vi "Info.vi"(9 "deutsch?":bool, 10 "virsualisierung?":bool, 11 "Version":string) -> ()   [LabVIEW 2012]
panel:
  in  "ende?":bool
  out "Numerisch":i32
  out "2D-Bild":picture
  out "Fehler (Ausgang)":errorcluster
  out "OK-Schaltfläche":bool
  # "2009 - 2011"
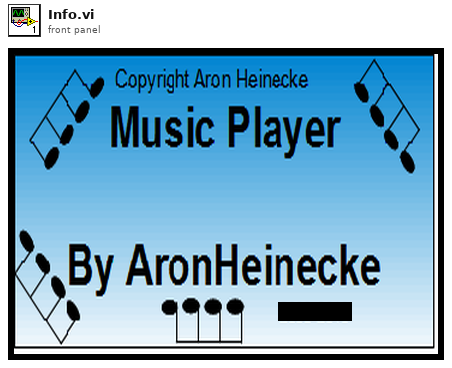
[diagram p1: front panel]
types:
  T1 = enum16{"None", "Stacked", "Clockwise", "Counterclockwise"}
  T2 = cluster{"Font Name:":string, "Size":i16, "Strikeout?":bool, "Italic?":bool, "Underline?":bool, "Outline?":bool, "Shadow?":bool, "Bold?":bool}
  T3 = cluster{"horizontal":enum16{"left", "center", "right"}, "vertical":enum16{"top", "center", "bottom"}}
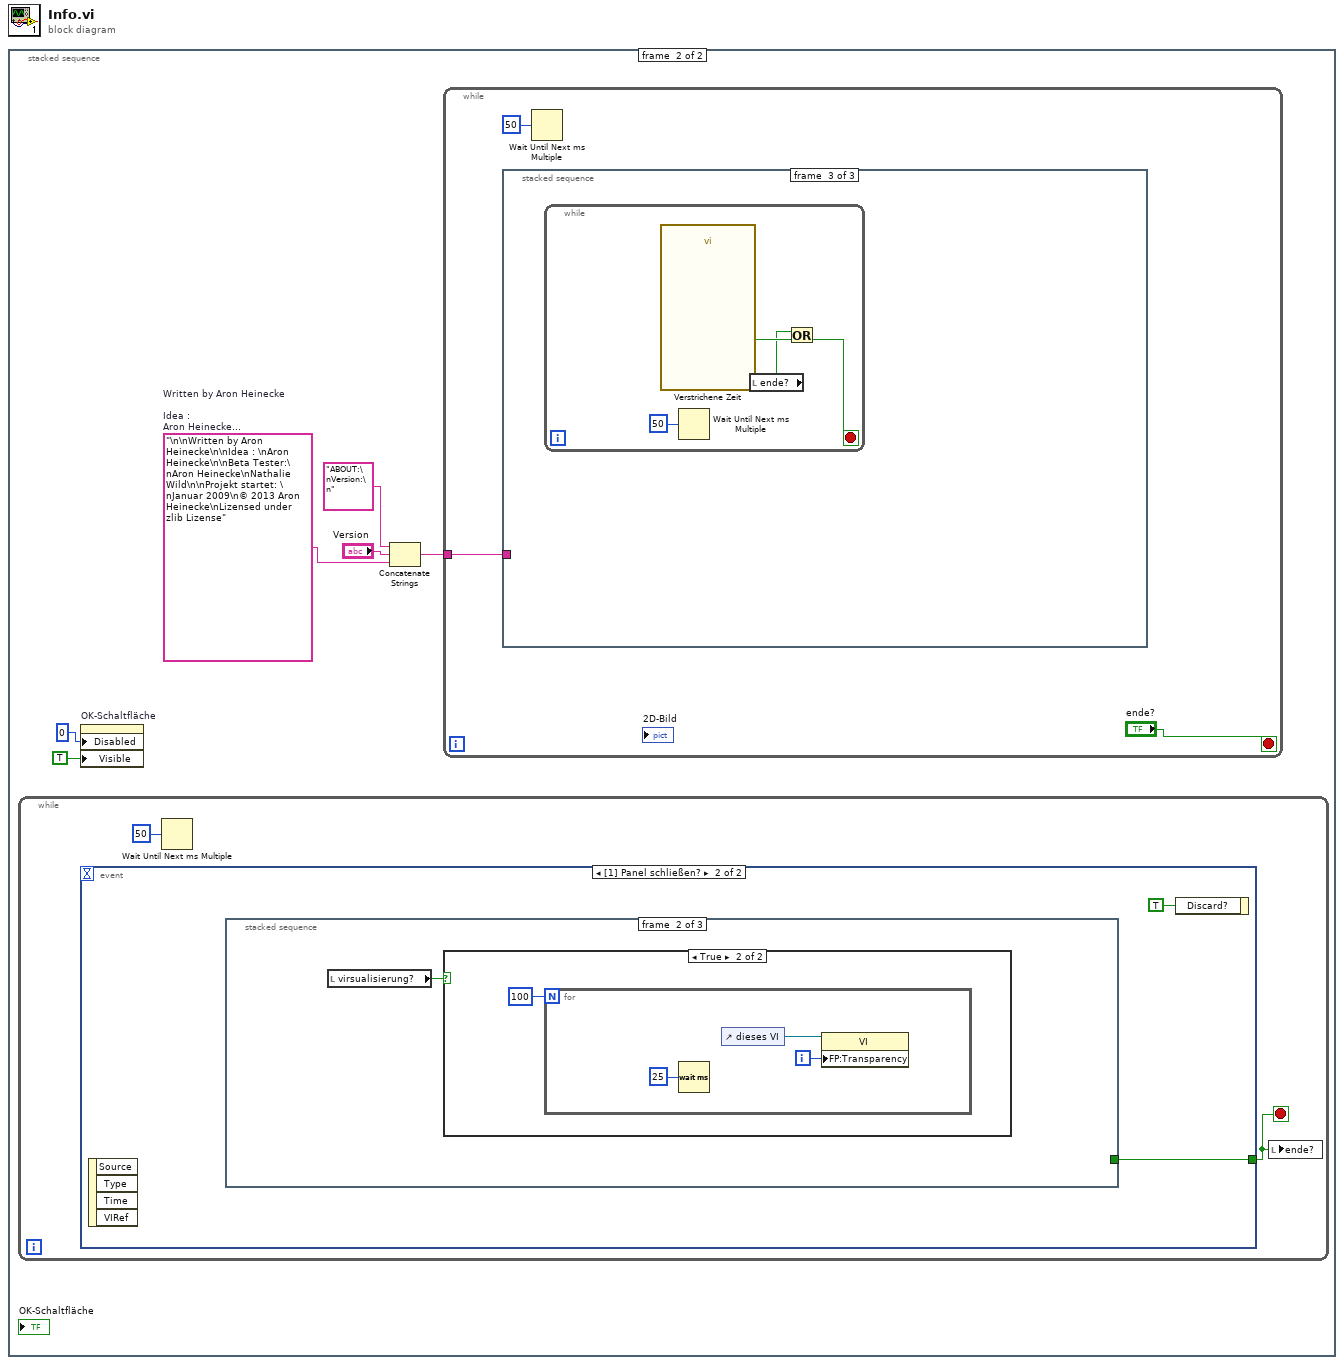
[diagram p0: block diagram]
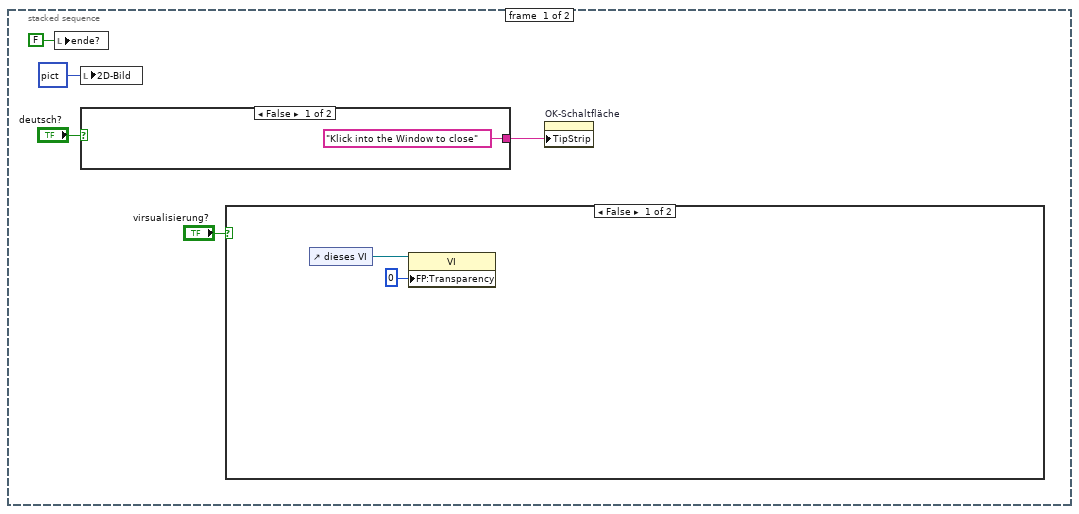
[diagram p2: hidden frame]
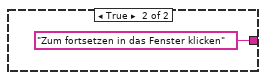
[diagram p3: hidden frame]
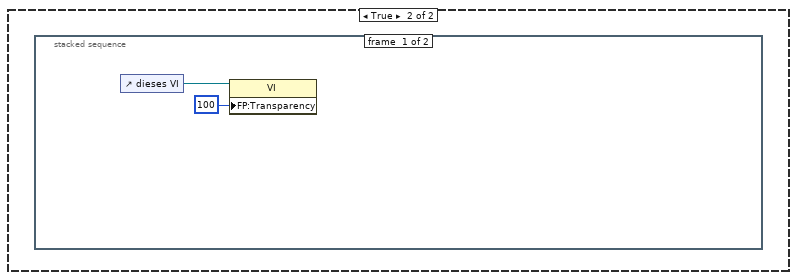
[diagram p4: hidden frame]
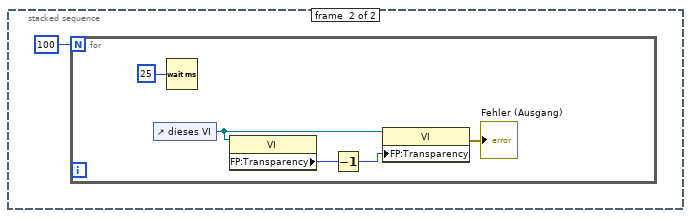
[diagram p5: hidden frame]
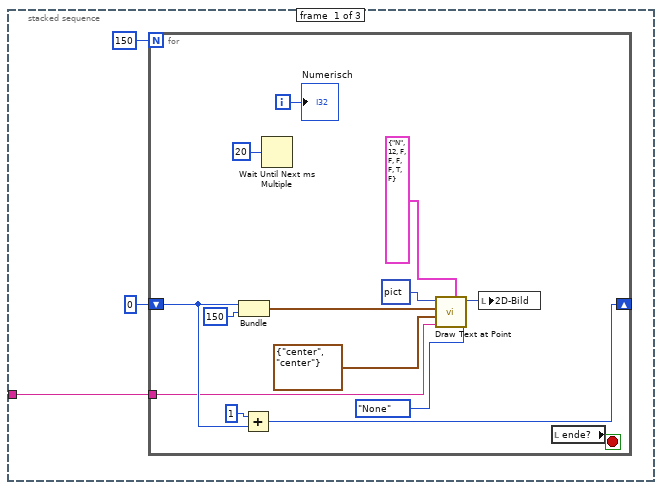
[diagram p6: hidden frame]
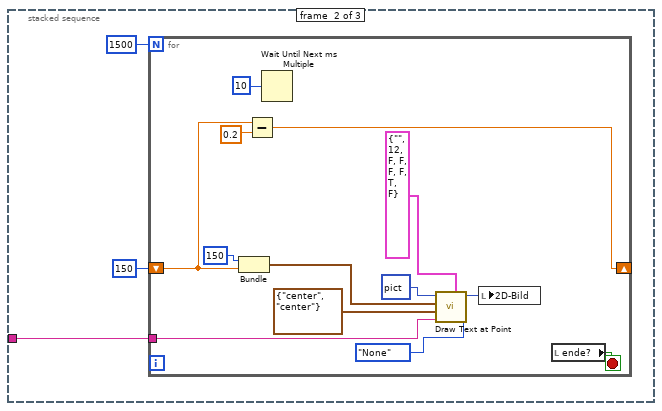
[diagram p7: hidden frame]
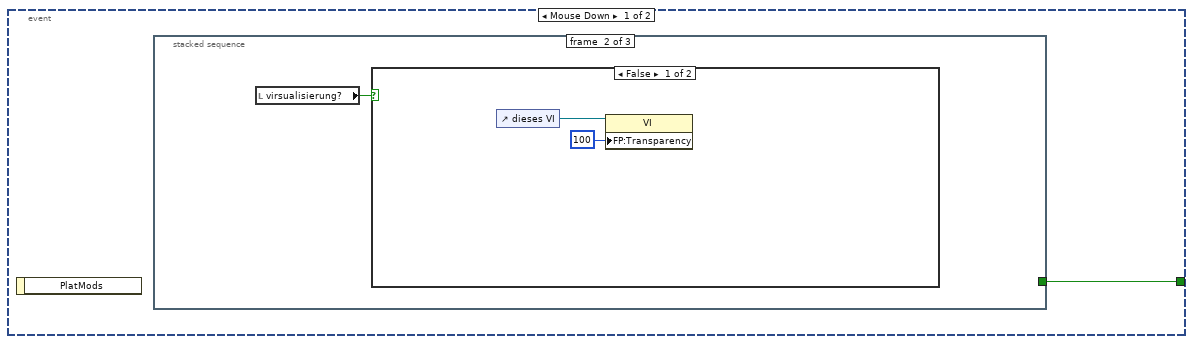
[diagram p8: hidden frame]
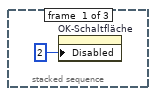
[diagram p9: hidden frame]
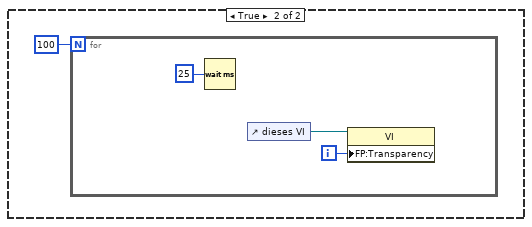
[diagram p10: hidden frame]
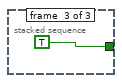
[diagram p11: hidden frame]
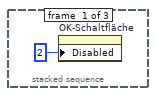
[diagram p12: hidden frame]
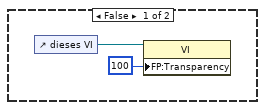
[diagram p13: hidden frame]
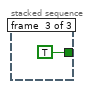
[diagram p14: hidden frame]
diagram:
  n1 = stacked-sequence {
    frame #0 {
      n2 = local write "ende?"(FALSE ("ende?")) -> ()
      n3 = local write "2D-Bild"(picture data[5B] ("2D-Bild")) -> ()
      n4 = case shown="False" "deutsch?" {
        tunnel: ["Klick into the Window to close" "Zum fortsetzen in das Fenster klicken"] -> w3
        frame False {
        }
        frame True {
        }
      }
      n5 = case shown="False" "virsualisierung?" {
        frame False {
          n6 = control-ref of="dieses VI"() -> (w9:refnum<vi>)
          n7 = property class="VI"(reference=w9, "FP:Transparency"=u8 0 ("Frontpanel-Fenster:Transparenz")) -> ()  [unwired: 1 in, 2 out]
        }
        frame True {
          n8 = stacked-sequence {
            frame #0 {
              n9 = control-ref of="dieses VI"() -> (w11:refnum<vi>)
              n10 = property class="VI"(reference=w11, "FP:Transparency"=u8 100 ("Frontpanel-Fenster:Transparenz")) -> ()  [unwired: 1 in, 2 out]
            }
            frame #1 {
              n11 = for {
                N: 100 -> [_]
                n12 = control-ref of="dieses VI"() -> (w17:refnum<vi>)
                n13 = Wait (ms)(milliseconds to wait=u32 25 ("Zu wartende ms")) -> ()  [unwired: 1 out]
                n14 = property class="VI"(reference=w17) -> ("FP:Transparency"=w16:u8)  [unwired: 1 in, 2 out]
                n15 = Decrement(x=w16) -> (x-1=w15:u8)
                n16 = property class="VI"(reference=w17, "FP:Transparency"=w15) -> (error out=→"Fehler (Ausgang)":errorcluster)  [unwired: 1 in, 1 out]
              }
            }
          }
        }
      }
      n17 = property on="OK-Schaltfläche" class="Bool."("TipStrip"=w3) -> ()  [unwired: 2 in, 2 out]
    }
    frame #1 {
      w20 = "\n\nWritten by Aron Heinecke\n\nIdea : \nAron Heinecke\n\nBeta Tester:\nAron Heinecke\nNathalie Wild\n\nProjekt startet: \nJanuar 2009\n© 2013 Aron Heinecke\nLizensed under zlib Lizense"  # Written by Aron Heinecke  Idea :  Aron Heinecke  Beta Tester: Aron Heinecke Nathalie Wild  Projekt startet:  Januar 2009 © 2013 Aron Heinecke Lizensed under zlib Lizense
      n18 = while {
        stop <- w64 stop-if-true
        n19 = event shown="[1] Panel schließen?" {
          selector: _ -> [_ _]
          dyn-events: _ -> [_ _]
          timeout: _ -> [_ _]
          tunnel: [w66 w76] -> w64
          event Mouse Down {
            n20 = event-data() -> ()  [unwired: 2 out]
            n21 = stacked-sequence {
              tunnel: [_ _ TRUE] -> w66
              frame #0 {
                n22 = property on="OK-Schaltfläche" class="Bool."("Disabled"=2) -> ()  [unwired: 2 in, 2 out]
              }
              frame #1 {
                n23 = local read "virsualisierung?"() -> (w68:bool)
                n24 = case shown="False" w68 {
                  frame False {
                    n25 = control-ref of="dieses VI"() -> (w70:refnum<vi>)
                    n26 = property class="VI"(reference=w70, "FP:Transparency"=u8 100 ("Frontpanel-Fenster:Transparenz")) -> ()  [unwired: 1 in, 2 out]
                  }
                  frame True {
                    n27 = for {
                      N: 100 -> [_]
                      i -> [w73]
                      n28 = Wait (ms)(milliseconds to wait=u32 25 ("Zu wartende ms")) -> ()  [unwired: 1 out]
                      n29 = control-ref of="dieses VI"() -> (w74:refnum<vi>)
                      n30 = property class="VI"(reference=w74, "FP:Transparency"=w73) -> ()  [unwired: 1 in, 2 out]
                    }
                  }
                }
              }
              frame #2 {
              }
            }
          }
          event Panel Close? {
            n31 = event-data() -> ()  [unwired: 5 out]
            n32 = stacked-sequence {
              tunnel: [_ _ TRUE] -> w76
              frame #0 {
                n33 = property on="OK-Schaltfläche" class="Bool."("Disabled"=u8 2 ("Deaktiviert")) -> ()  [unwired: 2 in, 2 out]
              }
              frame #1 {
                n34 = local read "virsualisierung?"() -> (w79:bool)
                n35 = case shown="True" w79 {
                  frame False {
                    n36 = control-ref of="dieses VI"() -> (w81:refnum<vi>)
                    n37 = property class="VI"(reference=w81, "FP:Transparency"=u8 100 ("Frontpanel-Fenster:Transparenz")) -> ()  [unwired: 1 in, 2 out]
                  }
                  frame True {
                    n38 = for {
                      N: 100 -> [_]
                      i -> [w84]
                      n39 = Wait (ms)(milliseconds to wait=u32 25 ("Zu wartende ms")) -> ()  [unwired: 1 out]
                      n40 = control-ref of="dieses VI"() -> (w85:refnum<vi>)
                      n41 = property class="VI"(reference=w85, "FP:Transparency"=w84) -> ()  [unwired: 1 in, 2 out]
                    }
                  }
                }
              }
              frame #2 {
              }
            }
            n42 = event-data("Discard?"=TRUE ("Verwerfen?")) -> ()  [unwired: 1 in, 1 out]
          }
        }
        n43 = Wait Until Next ms Multiple(millisecond multiple=50) -> ()  [unwired: 1 out]
        n44 = local write "ende?"(w64) -> ()
      }
      n45 = property on="OK-Schaltfläche" class="Bool."("Disabled"=0, "Visible"=TRUE) -> ()  [unwired: 2 in, 2 out]
      n46 = Concatenate Strings("ABOUT:\nVersion:\n", "Version", w20) -> (w18:string)
      n47 = while {
        tunnel: w18 -> [w25]
        stop <- "ende?" stop-if-true
        n48 = stacked-sequence {
          tunnel: w25 -> [w27 w44 _]
          frame #0 {
            n49 = for {
              N: 150 -> [_]
              shift-right: [w39] -> _
              shift-left: 0 -> [w40]
              tunnel: w27 -> [w31]
              i -> [w36]
              stop <- w32 stop-if-true
              n50 = Bundle(w40, 150) -> (w41:cluster{i32, i32})  [unwired: 1 in]
              n51 = Add(x=1, y=w40) -> (x+y=w39:i32)
              n52 = Wait Until Next ms Multiple(millisecond multiple=20) -> ()  [unwired: 1 out]
              n53 = call <vilib>:"Draw Text at Point.vi"("text orientation"=T1."None", "[user-specified font]"=T2 {"Font Name:"="N", "Size"=12, "Strikeout?"=FALSE, "Italic?"=FALSE, "Underline?"=FALSE, "Outline?"=FALSE, "Shadow?"=TRUE, "Bold?"=FALSE}, "text"=w31, "alignment(left, top)"=T3 {"horizontal"=enum."center", "vertical"=enum."center"}, "origin"=w41, "picture"=picture data[5B]) -> ("new picture"=w30:picture)  [unwired: 4 in, 1 out]
              n54 = local write "2D-Bild"(w30) -> ()
              n55 = local read "ende?"() -> (w32:bool)
              "Numerisch" <- w36
            }
          }
          frame #1 {
            n56 = for {
              N: 1500 -> [_]
              tunnel: w44 -> [w55]
              shift-right: [w50] -> _
              shift-left: 150 -> [w53]
              stop <- w47 stop-if-true
              n57 = Bundle(150, w53) -> (w52:cluster{i32, dbl})  [unwired: 1 in]
              n58 = Subtract(x=w53, y=0.2) -> (x-y=w50:dbl)
              n59 = Wait Until Next ms Multiple(millisecond multiple=10) -> ()  [unwired: 1 out]
              n60 = call <vilib>:"Draw Text at Point.vi"("text orientation"=T1."None", "[user-specified font]"=T2 {"Font Name:"="", "Size"=12, "Strikeout?"=FALSE, "Italic?"=FALSE, "Underline?"=FALSE, "Outline?"=FALSE, "Shadow?"=TRUE, "Bold?"=FALSE}, "text"=w55, "alignment(left, top)"=T3 {"horizontal"=enum."center", "vertical"=enum."center"}, "origin"=w52, "picture"=picture data[5B]) -> ("new picture"=w49:picture)  [unwired: 4 in, 1 out]
              n61 = local write "2D-Bild"(w49) -> ()
              n62 = local read "ende?"() -> (w47:bool)
            }
          }
          frame #2 {
            n63 = while {
              stop <- w61 stop-if-true
              n64 = call "Verstrichene Zeit"() -> ("Time has Elapsed"=w63:bool)  [unwired: 12 in, 7 out]
              n65 = Wait Until Next ms Multiple(millisecond multiple=u32 50 ("Vielfache von ms")) -> ()  [unwired: 1 out]
              n66 = local read "ende?"() -> (w60:bool)
              n67 = Or(x=w60, y=w63) -> (x .or. y?=w61:bool)
            }
          }
        }
        n68 = Wait Until Next ms Multiple(millisecond multiple=u32 50 ("Vielfache von ms")) -> ()  [unwired: 1 out]
      }
    }
  }
